vi "Read Config.vi"(8 "error in (no error)":errorcluster, 11 "Path":path) -> (0 "error out":errorcluster, 2 "Config":T1, 3 "File Created?":bool)   [LabVIEW 2020, in "VI Properties Editor.lvlib"]
doc: "Reads a config file located at <B>Path</B>."
uses:
  VI Properties Editor.lvlib
  <vilib>/Utility/config.llb/NI_LVConfig.lvlib
  <vilib>/Utility/config.llb/Read Key (Boolean).vi
  CTLs/Config.ctl
  <vilib>/Utility/config.llb/Read Key (String).vi
  CTLs/Filter Type.ctl
  CTLs/Column Name.ctl
  CTLs/Filter Info.ctl
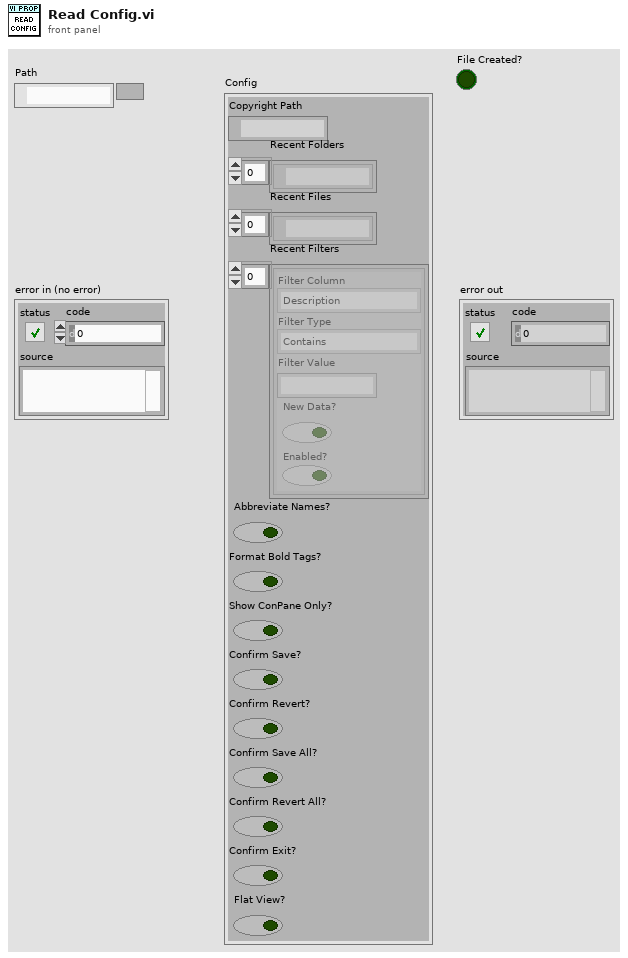
[diagram p1: front panel]
types:
  T1 = typedef "VI Properties Editor.lvlib/Config.ctl" = cluster{"Copyright Path":path, "Recent Folders":path[], "Recent Files":path[], "Recent Filters":T2[], "Abbreviate Names?":bool, "Format Bold Tags?":bool, "Show ConPane Only?":bool, "Confirm Save?":bool, "Confirm Revert?":bool, "Confirm Save All?":bool, "Confirm Revert All?":bool, "Confirm Exit?":bool, "Flat View?":bool}
  T2 = typedef "VI Properties Editor.lvlib/Filter Info.ctl" = cluster{"Filter Column":T3, "Filter Type":T4, "Filter Value":string, "New Data?":bool, "Enabled?":bool}
  T3 = typedef "VI Properties Editor.lvlib/Column Name.ctl" = enum16{"Name", "Path", "Type", "Window Title", "Description", "Help Path", "Help Tag", "Custom Title?", "Reentrancy", "Inlined?", "Help URL", "Help Type", "Allow Debugging?", "Auto Error Handling?", "Run When Opened?", "Suspend When Called?", "Priority", "Preferred Exec Sytem"}
  T4 = typedef "VI Properties Editor.lvlib/Filter Type.ctl" = enum16{"Contains", "Equals", "Starts with", "Ends with", "Does not contain", "Does not equal", "Is empty", "Is not empty"}
  T5 = typedef "NI_LVConfig.lvlib/Config Data RefNum.ctl" = refnum<k1>
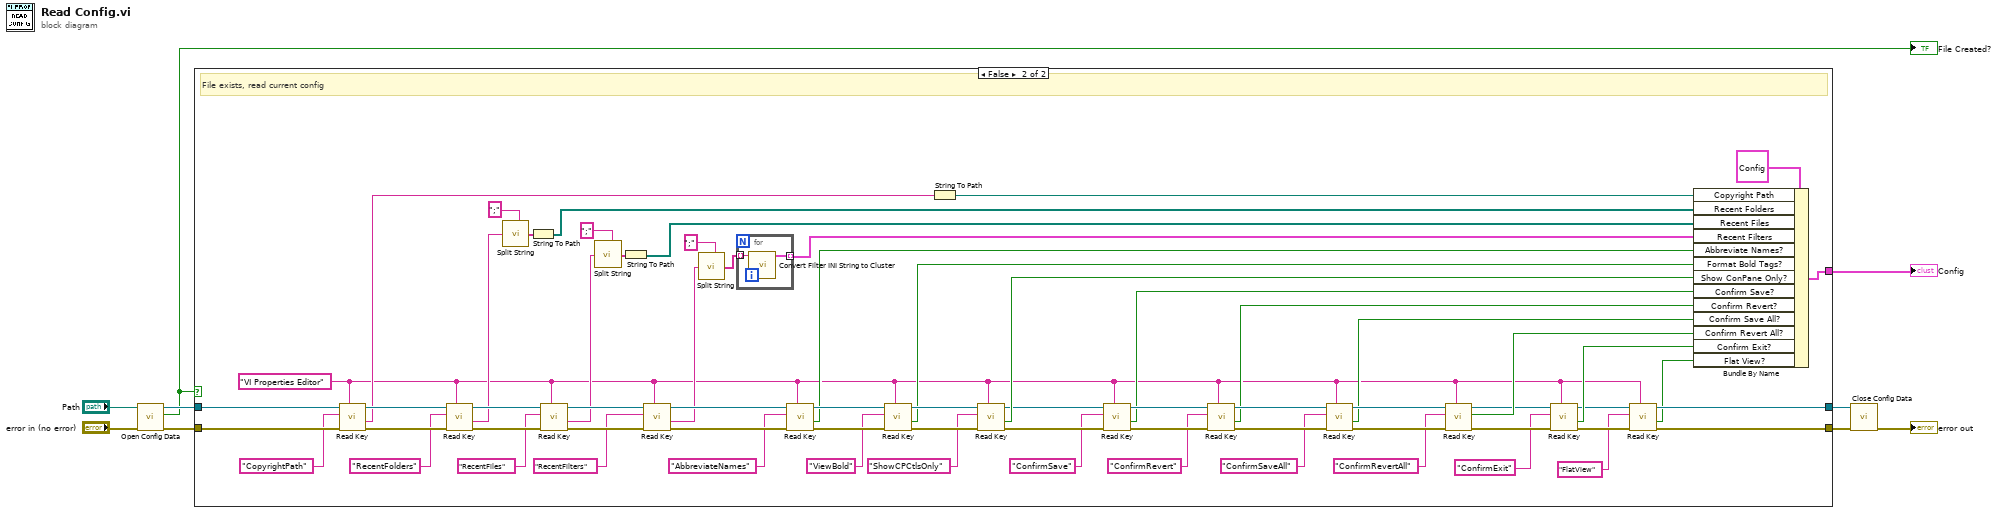
[diagram p0: block diagram]
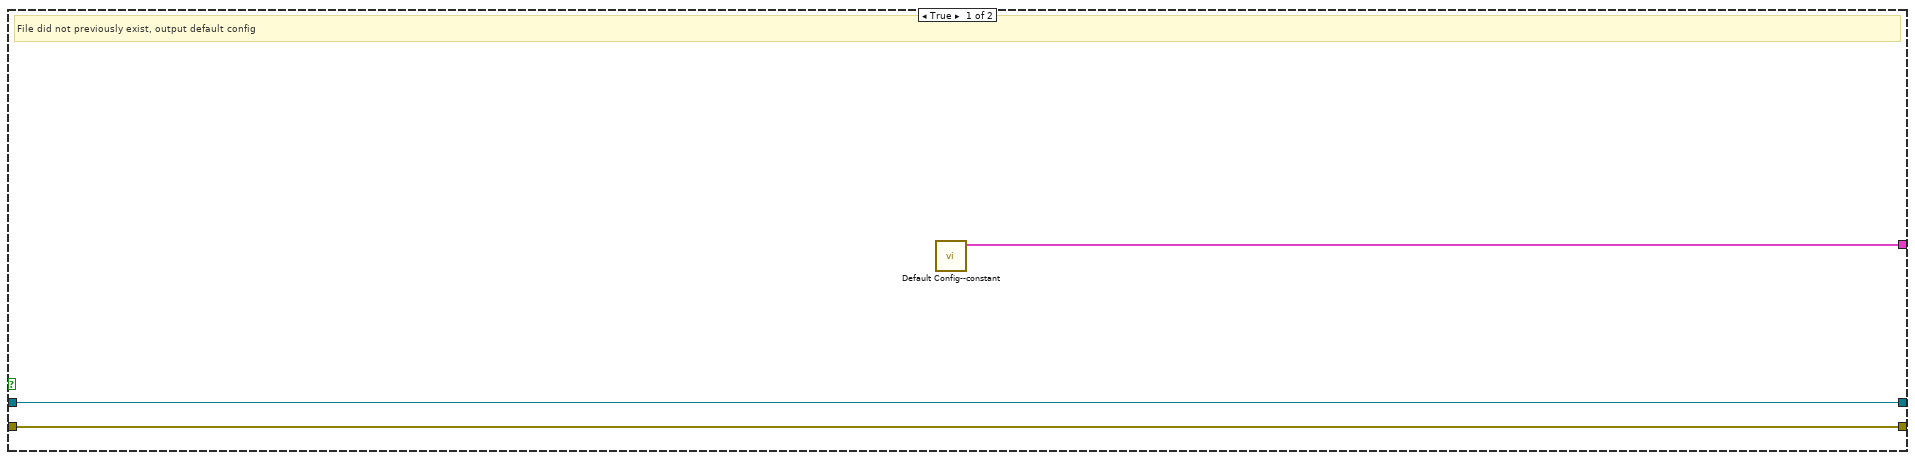
[diagram p2: hidden frame]
diagram:
  n1 = call <vilib>:"Open Config Data.vi"("error in (no error)"="error in (no error)", "configuration file path"="Path") -> ("error out"=w8:errorcluster, "file created?"=w2:bool, "refnum"=w4:T5)  [unwired: 7 in]
  "File Created?" <- w2
  n2 = case shown="False" w2 {
    tunnel: w4 -> [w10 w63]
    tunnel: w8 -> [w12 w76]
    tunnel: [w12 w18] -> w7
    tunnel: [w10 w16] -> w3
    tunnel: [w11 w56] -> w1
    frame True {
      # "File did not previously exist, output default config"
      n3 = call "Default Config--constant.vi"() -> ("Default Config"=w11:T1)  [unwired: 11 in]
    }
    frame False {
      w15 = "VI Properties Editor" ("section")
      # "File exists, read current config"
      n4 = call-poly <vilib>:"Read Key.vi"("section"=w15, "error in (no error)"=w76, "key"="CopyrightPath", "refnum"=w63) -> ("error out"=w73:errorcluster, "value"=w55:string, "refnum out"=w65:T5)  [unwired: 4 in, 1 out]
      n5 = call-poly <vilib>:"Read Key.vi"("section"=w15, "error in (no error)"=w73, "key"="RecentFolders", "refnum"=w65) -> ("error out"=w72:errorcluster, "value"=w49:string, "refnum out"=w64:T5)  [unwired: 4 in, 1 out]
      n6 = call <vilib>:"Split String.vi"("Split Pattern"=";", "Input String"=w49) -> ("Split String"=w48:string[])  [unwired: 5 in]
      n7 = String To Path(string=w48) -> (path=w47:path[])
      n8 = call-poly <vilib>:"Read Key.vi"("section"=w15, "error in (no error)"=w72, "key"="RecentFiles", "refnum"=w64) -> ("error out"=w71:errorcluster, "value"=w44:string, "refnum out"=w77:T5)  [unwired: 4 in, 1 out]
      n9 = call <vilib>:"Split String.vi"("Split Pattern"=";", "Input String"=w44) -> ("Split String"=w46:string[])  [unwired: 5 in]
      n10 = String To Path(string=w46) -> (path=w43:path[])
      n11 = call-poly <vilib>:"Read Key.vi"("section"=w15, "error in (no error)"=w71, "key"="RecentFilters", "refnum"=w77) -> ("error out"=w78:errorcluster, "value"=w25:string, "refnum out"=w28:T5)  [unwired: 4 in, 1 out]
      n12 = call <vilib>:"Split String.vi"("Split Pattern"=";", "Input String"=w25) -> ("Split String"=w24:string[])  [unwired: 5 in]
      n13 = for {
        tunnel: w24 -> [w81] mode=indexing
        tunnel: [w80] -> w23 mode=indexing
        n14 = call "Convert Filter INI String to Cluster.vi"("INI String"=w81) -> ("Filter Info"=w80:T2)  [unwired: 10 in]
      }
      n15 = call-poly <vilib>:"Read Key.vi"("section"=w15, "error in (no error)"=w78, "key"="AbbreviateNames", "refnum"=w28) -> ("error out"=w75:errorcluster, "value"=w54:bool, "refnum out"=w60:T5)  [unwired: 4 in, 1 out]
      n16 = call-poly <vilib>:"Read Key.vi"("section"=w15, "error in (no error)"=w75, "key"="ViewBold", "refnum"=w60) -> ("error out"=w74:errorcluster, "value"=w53:bool, "refnum out"=w66:T5)  [unwired: 4 in, 1 out]
      n17 = String To Path(string=w55) -> (path=w58:path)
      n18 = call-poly <vilib>:"Read Key.vi"("section"=w15, "error in (no error)"=w74, "key"="ShowCPCtlsOnly", "refnum"=w66) -> ("error out"=w68:errorcluster, "value"=w41:bool, "refnum out"=w36:T5)  [unwired: 4 in, 1 out]
      n19 = call-poly <vilib>:"Read Key.vi"("section"=w15, "error in (no error)"=w68, "key"="ConfirmSave", "refnum"=w36) -> ("error out"=w70:errorcluster, "value"=w32:bool, "refnum out"=w35:T5)  [unwired: 4 in, 1 out]
      n20 = call-poly <vilib>:"Read Key.vi"("section"=w15, "error in (no error)"=w70, "key"="ConfirmRevert", "refnum"=w35) -> ("error out"=w67:errorcluster, "value"=w31:bool, "refnum out"=w34:T5)  [unwired: 4 in, 1 out]
      n21 = call-poly <vilib>:"Read Key.vi"("section"=w15, "error in (no error)"=w67, "key"="ConfirmSaveAll", "refnum"=w34) -> ("error out"=w69:errorcluster, "value"=w30:bool, "refnum out"=w33:T5)  [unwired: 4 in, 1 out]
      n22 = call-poly <vilib>:"Read Key.vi"("section"=w15, "error in (no error)"=w69, "key"="ConfirmRevertAll", "refnum"=w33) -> ("error out"=w79:errorcluster, "found?"=w29:bool, "refnum out"=w21:T5)  [unwired: 4 in, 1 out]
      n23 = call-poly <vilib>:"Read Key.vi"("section"=w15, "error in (no error)"=w79, "key"="ConfirmExit", "refnum"=w21) -> ("error out"=w20:errorcluster, "value"=w19:bool, "refnum out"=w17:T5)  [unwired: 4 in, 1 out]
      n24 = call-poly <vilib>:"Read Key.vi"("section"=w15, "error in (no error)"=w20, "key"="FlatView", "refnum"=w17) -> ("error out"=w18:errorcluster, "value"=w13:bool, "refnum out"=w16:T5)  [unwired: 4 in, 1 out]
      n25 = Bundle By Name(cluster=T1 {"Copyright Path"=path "", "Recent Folders"=[], "Recent Files"=[], "Recent Filters"=[], "Abbreviate Names?"=FALSE, "Format Bold Tags?"=FALSE, "Show ConPane Only?"=FALSE, "Confirm Save?"=FALSE, "Confirm Revert?"=FALSE, "Confirm Save All?"=FALSE, "Confirm Revert All?"=FALSE, "Confirm Exit?"=FALSE, "Flat View?"=FALSE} ("Config"), "Copyright Path"=w58, "Recent Folders"=w47, "Recent Files"=w43, "Recent Filters"=w23, "Abbreviate Names?"=w54, "Format Bold Tags?"=w53, "Show ConPane Only?"=w41, "Confirm Save?"=w32, "Confirm Revert?"=w31, "Confirm Save All?"=w30, "Confirm Revert All?"=w29, "Confirm Exit?"=w19, "Flat View?"=w13) -> (w56:T1)
    }
  }
  "Config" <- w1
  n26 = call <vilib>:"Close Config Data.vi"("error in (no error)"=w7, "refnum"=w3) -> ("error out"=→"error out":errorcluster)  [unwired: 8 in, 1 out]
